vi "conversion_deg_to_rpm.vi"(1 "x (deg/s)":dbl) -> (0 "x (rpm)":dbl)   [LabVIEW 2021]
doc: "Converts deg/s to rpm."
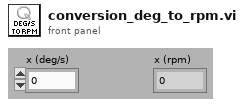
[diagram p1: front panel]
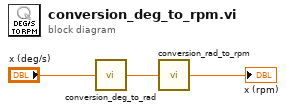
[diagram p0: block diagram]
diagram:
  n1 = call "conversion_deg_to_rad.vi"("Angle (deg)"="x (deg/s)") -> ("Angle (rad)"=w1:dbl)
  n2 = call "conversion_rad_to_rpm.vi"("x (rad/s)"=w1) -> ("x (rpm)"=→"x (rpm)":dbl)
